vi "PID (Compatibility).vi"(4 "iteration":i32, 6 "options":T1={"sp low"=0.0, "sp high"=100.0, "out low"=-100.0, "out high"=100.0, "hold (F)"=FALSE, "auto (T)"=TRUE, "pro. band (F)"=FALSE, "reverse acting (T)"=TRUE, "beta"=1.0, "linearity"=1.0, "dt (s)"=-1.0} {"dt (s)" format="%.2f"; "linearity" min=0.0 max=1.0 format="%.2f"; "sp low" format="%.2f"; "sp high" format="%.2f"; "out low" format="%.2f"; "out high" format="%.2f"; "beta" min=0.0 max=1.0 format="%.2f"}, 8 "manual control":dbl format="%.2f", 9 "PID parameters":cluster{"Kp":dbl, "Ti":dbl, "Td":dbl} {"Td" format="%.2f"; "Ti" format="%.2f"; "Kp" format="%.2f"}, 10 "process variable":dbl format="%.2f", 11 "setpoint":dbl format="%.2f") -> (3 "output":dbl format="%.2f")   [LabVIEW 2012]
doc: "Description of the PID algorithm:\n\nDerivative action is on the process variable only. Anti-reset windup and bumpless transfer are supported.\n\nThis VI should be called from inside a while loop with a fixed cycle time. If Cycle Time is less than or equal to zero, an internal timer with 1 millisecond resolution is used for calculations.\n\nThis VI is reentrant, so you can call it from multiple, independent higher-level VIs without interference.\n\nThe default variable ranges correspond to setpoint, process variable, and output expressed in percent. Reverse action (also called increase-decrease) is the \"normal\" controller mode where the output decreases if the process variable is higher than the setpoint.\n\nSwitching from auto to manual is bumpless; the initial value of the Manual Output control is subtracted out so that it is really a \"relative\" output control. Switching from manual to auto is also bumpless.\n\nSwitching to Hold causes the controller to ignore further changes in the process variable and suspends any integral action. Thus, the output stays constant at the last value."
uses:
  Auto/manual.vi
panel:
  # "hold (F): default FALSE, no hold.\nauto (T): default TRUE, PID controlling.\npro.band(F): default FALSE, Gain is expressed in actual gain.\n     if TRUE, the proportional band is used.  The relationship \n     between proportional band and gain is gain=100/pro. band\nreverse acting (T): default TRUE, reverse acting. In reverse \n     acting, controller output increases when sp-pv increases.\nsp & pv range: setpoint and process variable range.  Can\n     be either in percentage or actual engineering units.\noutput range: controller output range.  Can be either in\n     percentage or actual engineering units.\nbeta: default 1.0. smaller beta reduces the overshoot in   \n     setpoint response.\nmanual control: when auto is FALSE, controller output =\n     manual control.\nlinearity: default 1.0, linear control action. smaller value \n     reduces controller gain when PV is close to SP."
  # "PID Controller"
  # "SP & PV range:"
  # "Output range:"
  # "-1: default,using\nsystem clock"
  # "Proportional gain or band (Kc)"
  # "Integral (reset) time (Ti, min)"
  # "Derivative (rate) time (Td, min)"
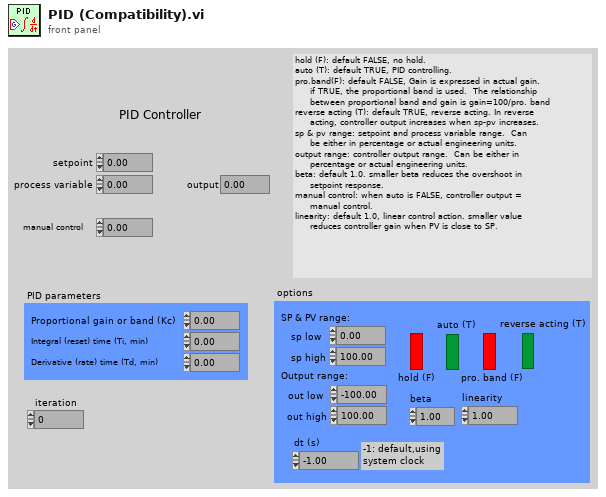
[diagram p1: front panel]
types:
  T1 = cluster{"sp low":dbl, "sp high":dbl, "out low":dbl, "out high":dbl, "hold (F)":bool, "auto (T)":bool, "pro. band (F)":bool, "reverse acting (T)":bool, "beta":dbl, "linearity":dbl, "dt (s)":dbl}
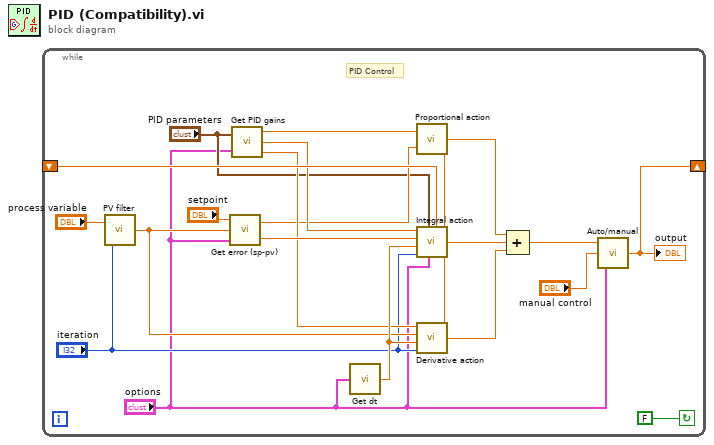
[diagram p0: block diagram]
diagram:
  n1 = while {
    shift-left: _ -> [w20]
    shift-right: [w6] -> _
    stop <- FALSE continue-if-true
    # "PID Control"
    n2 = call "PV filter.vi"("iteration"="iteration", "process variable"="process variable") -> ("filtered pv"=w15:dbl)
    n3 = call "Get error (sp-pv).vi"("options"="options", "process variable"=w15, "setpoint"="setpoint") -> ("error"=w14:dbl, "error (with beta)"=w10:dbl)
    n4 = call "Get PID gains.vi"("PID parameters"="PID parameters", "options"="options") -> ("Kc"=w11:dbl, "Ki"=w12:dbl, "Kd"=w13:dbl)
    n5 = call "Get dt.vi"("options"="options") -> ("dt (min.)"=w16:dbl)
    n6 = call "Proportional action.vi"("error"=w10, "Kc"=w11) -> ("proportional action"=w19:dbl)
    n7 = call "Derivative action.vi"("iteration"="iteration", "dt"=w16, "process variable"=w15, "Kd"=w13) -> ("derivative action"=w18:dbl)
    n8 = call "Integral action.vi"("derivative action"=w18, "proportional action"=w19, "prev. control output"=w20, "options"="options", "PID parameters"="PID parameters", "iteration"="iteration", "dt"=w16, "error"=w14, "Ki"=w12) -> ("integral action"=w17:dbl)  [unwired: 2 in]
    n9 = Compound Arithmetic op=ADD(w19, w17, w18) -> (w8:dbl)
    n10 = call "Auto/manual.vi"("options"="options", "manual control"="manual control", "auto control"=w8) -> ("output"=w6:dbl)
    "output" <- w6
  }
